vi "Report App Info.vi"(8 "error in (no error)":errorcluster, 11 "Volatus Core in":refnum<class "Volatus Core.lvclass">) -> (0 "error out":errorcluster, 3 "Volatus Core out":refnum<class "Volatus Core.lvclass">)   [LabVIEW 2020, in "Volatus.lvlib" / "Volatus Core.lvclass"]
uses:
  Volatus Core.lvclass
  Volatus Core.lvclass/Volatus Core.ctl
  Module/Module.lvclass
  lv-vecto/Vecto/Node Config/Node Config.lvclass
  C:/dev/lv20CE/relink/lv-volatus/Volatus/Module/Module.lvclass
  C:/dev/lv20CE/relink/lv-volatus/Volatus/Volatus Core/Volatus Core.lvclass
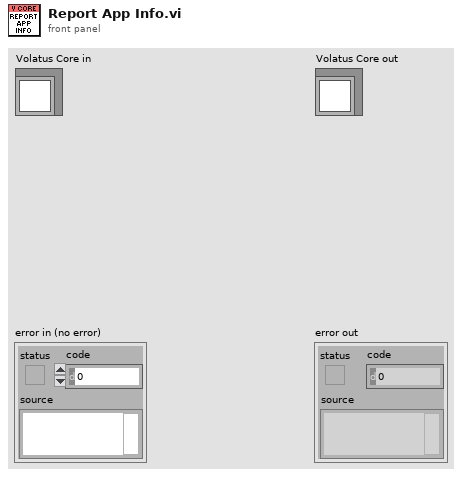
[diagram p1: front panel]
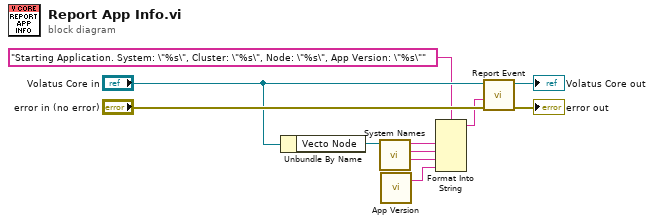
[diagram p0: block diagram]
diagram:
  n1 = Unbundle By Name("Volatus Core in") -> ("Vecto Node"=w4:refnum<class "Node Config.lvclass">)
  n2 = call "System Names.vi"("Node Config in"=w4) -> ("Name"=w1:string, "Cluster"=w2:string, "System"=w3:string)  [unwired: 8 in]
  n3 = call "App Version.vi"() -> ("App Version"=w6:string)  [unwired: 3 in]
  n4 = Format Into String(format string="Starting Application. System: \"%s\", Cluster: \"%s\", Node: \"%s\", App Version: \"%s\"", w3, w2, w1, w6) -> (resulting string=w8:string)  [unwired: 2 in, 1 out]
  n5 = call "Report Event.vi"("error in (no error)"="error in (no error)", "Message"=w8, "Module in"="Volatus Core in") -> ("error out"=→"error out":errorcluster, "Module out"=→"Volatus Core out":refnum<class "Volatus Core.lvclass">)  [unwired: 7 in]
